vi "UpdateServerErrorStatus.vi"(10 "Error":string="1") -> ()   [LabVIEW 2011]
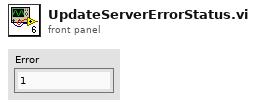
[diagram p1: front panel]
types:
  T1 = enum16{"open", "replace", "create", "open or create", "replace or create", "replace or create with confirmation"}
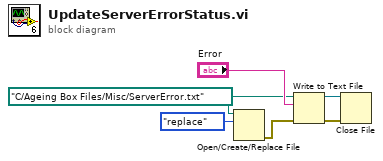
[diagram p0: block diagram]
diagram:
  w2 = path "C:/Ageing Box Files/Misc/ServerError.txt" ("file path (use dialog)")
  n1 = Open/Create/Replace File(file path (use dialog)=w2, operation (0:open)=T1."replace") -> (error out=w3:errorcluster)  [unwired: 4 in, 2 out]
  n2 = Write to Text File(file (use dialog)=w2, text="Error", error in=w3) -> (refnum out=w6:refnum<file>, error out=w5:errorcluster)  [unwired: 1 in, 1 out]
  n3 = Close File(refnum=w6, error in=w5) -> ()  [unwired: 2 out]
